vi "Set Cell Bg Colour.vi"(8 "Column":i32=-1, 9 "Row":i32=-1, 10 "Color Box":u32(colorbox)=13816530, 11 "Excel Sheet in":refnum<class "Excel Sheet.lvclass">) -> (3 "Excel Sheet out":refnum<class "Excel Sheet.lvclass">)   [LabVIEW 2016, in "Excel Sheet.lvclass"]
uses:
  Excel Sheet.lvclass
panel:
  out "error out":errorcluster
  in  "error in (no error)":errorcluster
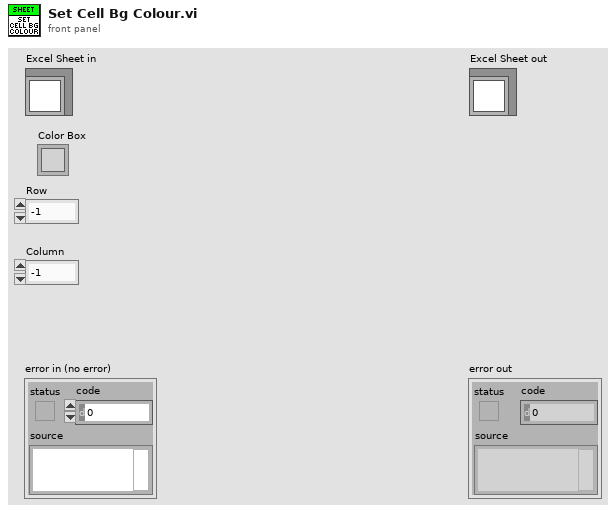
[diagram p1: front panel]
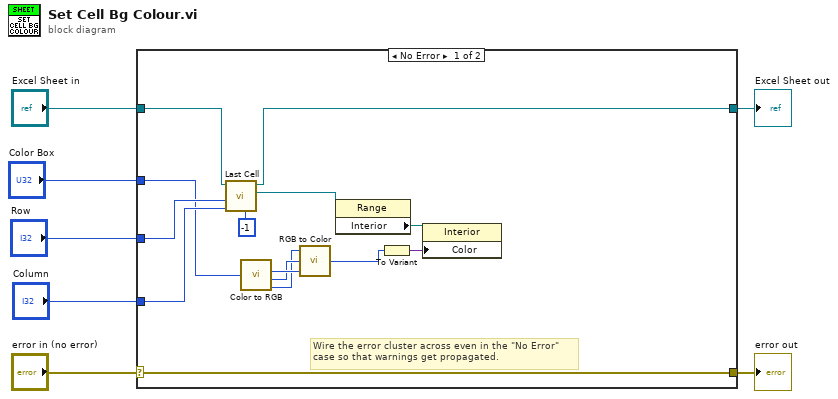
[diagram p0: block diagram]
diagram:
  n1 = case shown="No Error" "error in (no error)" {
    selector: "error in (no error)" -> [w21 w23]
    tunnel: [w21 w23] -> w6
    tunnel: [w19 w22] -> w4
    tunnel: "Excel Sheet in" -> [w20 w22]
    tunnel: "Color Box" -> [w10 _]
    tunnel: "Column" -> [w15 _]
    tunnel: "Row" -> [w14 _]
    frame No Error {
      # "Wire the error cluster across even in the \"No Error\"\ncase so that warnings get propagated."
      n2 = call "Last Cell.vi"("Col Offset"=-1, "Column"=w15, "Row"=w14, "Excel Sheet in"=w20) -> ("Cell"=w17:refnum<k7>, "Excel Sheet out"=w19:refnum<class "Excel Sheet.lvclass">)  [unwired: 4 in, 2 out]
      n3 = call <vilib>:"Color to RGB.vi"("Color"=w10) -> ("R"=w13:u8, "G"=w12:u8, "B"=w11:u8)  [unwired: 1 out]
      n4 = call <vilib>:"RGB to Color.vi"("B"=w13, "G"=w12, "R"=w11) -> ("Color"=w8:u32)
      n5 = property class="Range"(reference=w17) -> ("Interior"=w16:refnum<k7>)  [unwired: 1 in, 2 out]
      n6 = To Variant(anything=w8) -> (Variant=w9:variant)
      n7 = property class="Interior"(reference=w16, "Color"=w9) -> ()  [unwired: 1 in, 2 out]
    }
    frame Error {
    }
  }
  "error out" <- w6
  "Excel Sheet out" <- w4
